vi "NET_Drive_Cluster.vi"(8 "Read(F) Write(T)":bool=TRUE, 11 "CMD_DriveCluster":T1) -> (3 "CMD_DriveCluster Out":T1)   [LabVIEW 2017]
uses:
  RoboRio Code/TypeDef/CLUSTER_CMD_WC_Drive.ctl
  RoboRio Code/TypeDef/ENUM_WC_Drive_DriveMode.ctl
  RoboRio Code/TypeDef/CLUSTER_Drive_ACT Loop_VBus Data.ctl
  RoboRio Code/TypeDef/CLUSTER_X and Y.ctl
  RoboRio Code/TypeDef/CLUSTER_Drive_ACT Loop_Profile Data.ctl
  <vilib>/Rock Robotics/Network Tables/NT Read Numeric Array.vi
  <vilib>/Rock Robotics/Network Tables/NT Read Boolean.vi
  <vilib>/Rock Robotics/Network Tables/NT Read Number.vi
  <vilib>/Rock Robotics/Network Tables/NT Write Numeric Array.vi
  <vilib>/Rock Robotics/Network Tables/NT Write Boolean.vi
  <vilib>/Rock Robotics/Network Tables/NT Write Number.vi
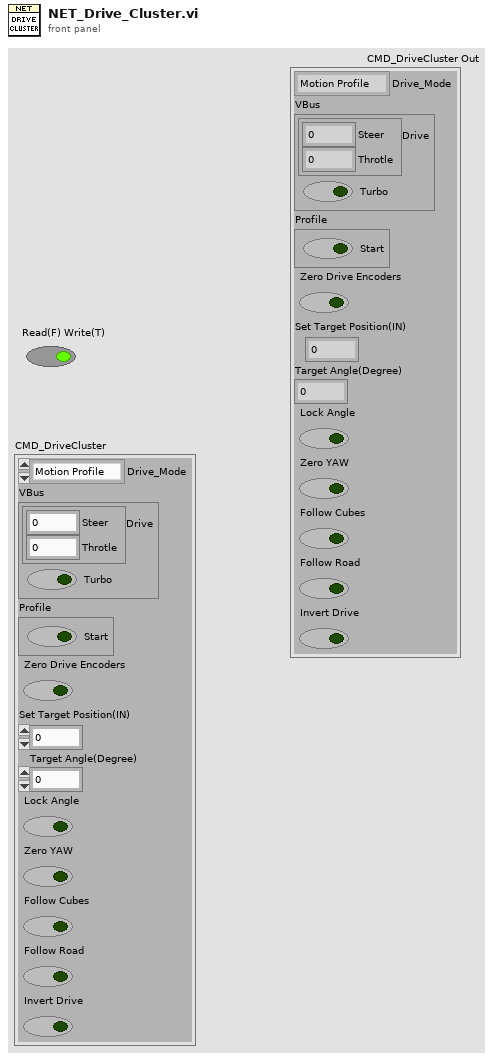
[diagram p1: front panel]
types:
  T1 = typedef "CLUSTER_CMD_WC_Drive.ctl" = cluster{"Drive_Mode":T2, "VBus":T3, "Profile":T5, "Zero Drive Encoders":bool, "Set Target Position(IN)":dbl, "Target Angle(Degree)":dbl, "Lock Angle":bool, "Zero YAW":bool, "Follow Cubes":bool, "Follow Road":bool, "Invert Drive":bool}
  T2 = typedef "ENUM_WC_Drive_DriveMode.ctl" = enum16{"Motion Profile", "CrossLineAuto", "VBus", "Stop"}
  T3 = typedef "CLUSTER_Drive_ACT Loop_VBus Data.ctl" = cluster{"Drive":T4, "Turbo":bool}
  T4 = typedef "CLUSTER_X and Y.ctl" = cluster{"Steer":dbl, "Throtle":dbl}
  T5 = typedef "CLUSTER_Drive_ACT Loop_Profile Data.ctl" = cluster{"Start":bool}
  T6 = cluster{"Numeric Array[0]":dbl, "Numeric Array[1]":dbl}
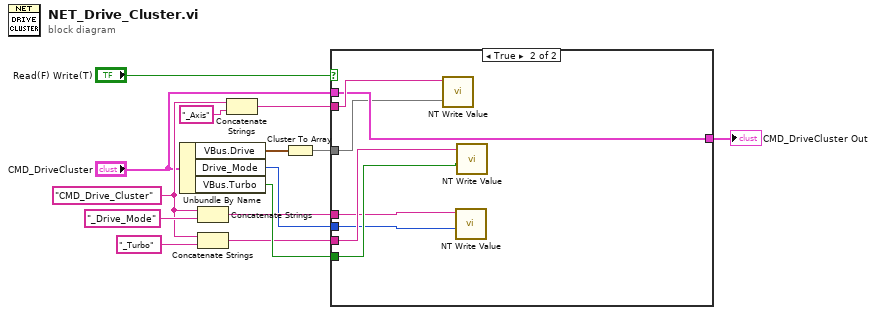
[diagram p0: block diagram]
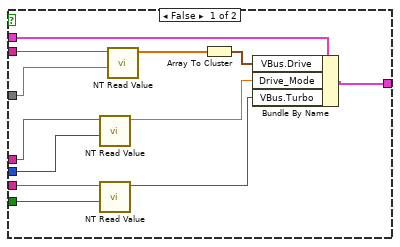
[diagram p2: hidden frame]
diagram:
  w7 = "CMD_Drive_Cluster" ("Name")
  n1 = Unbundle By Name("CMD_DriveCluster") -> ("VBus.Drive"=w3:T4, "Drive_Mode"=w1:T2, "VBus.Turbo"=w13:bool)
  n2 = Concatenate Strings(w7, "_Drive_Mode" ("string")) -> (w8:string)
  n3 = Concatenate Strings(w7, "_Turbo" ("string")) -> (w5:string)
  n4 = Concatenate Strings(w7, "_Axis" ("string")) -> (w10:string)
  n5 = Cluster To Array(cluster=w3) -> (array=w2:dbl[])
  n6 = case shown="True" "Read(F) Write(T)" {
    tunnel: w1 -> [w16 w27]
    tunnel: w13 -> [w26 w29]
    tunnel: [w17 w32] -> w12
    tunnel: w10 -> [w25 w33]
    tunnel: w8 -> [w24 w28]
    tunnel: w5 -> [w23 w30]
    tunnel: "CMD_DriveCluster" -> [w22 w32]
    tunnel: w2 -> [w18 w31]
    frame False {
      n7 = call-poly <vilib>:"NT Read Value.vi"("Default Value"=w16, "Name"=w24) -> ("Numeric"=w15:dbl)  [unwired: 8 in, 1 out]
      n8 = call-poly <vilib>:"NT Read Value.vi"("Default Value"=w26, "Name"=w23) -> ("Boolean"=w21:bool)  [unwired: 8 in, 1 out]
      n9 = call-poly <vilib>:"NT Read Value.vi"("Default Value"=w18, "Name"=w25) -> ("Numeric Array"=w20:dbl[])  [unwired: 8 in, 1 out]
      n10 = Array To Cluster(array=w20) -> (cluster=w19:T6)
      n11 = Bundle By Name(cluster=w22, "VBus.Drive"=w19, "Drive_Mode"=w15, "VBus.Turbo"=w21) -> (w17:T1)
    }
    frame True {
      n12 = call-poly <vilib>:"NT Write Value.vi"("Numeric Array"=w31, "Name"=w33) -> ()  [unwired: 9 in, 1 out]
      n13 = call-poly <vilib>:"NT Write Value.vi"("Numeric"=w27, "Name"=w28) -> ()  [unwired: 9 in, 1 out]
      n14 = call-poly <vilib>:"NT Write Value.vi"("Boolean"=w29, "Name"=w30) -> ()  [unwired: 9 in, 1 out]
    }
  }
  "CMD_DriveCluster Out" <- w12
